vi "Read Started.vi"(8 "error in (no error)":errorcluster, 11 "MQTT_Base in":refnum<class "MQTT_Base.lvclass">) -> (0 "error out":errorcluster, 2 "Started":refnum<notifier>, 3 "MQTT_Base out":refnum<class "MQTT_Base.lvclass">)   [LabVIEW 2013, in "MQTT Base.lvlib" / "MQTT_Base.lvclass"]
uses:
  MQTT_Base.lvclass
  MQTT_Base.lvclass/MQTT_Base.ctl
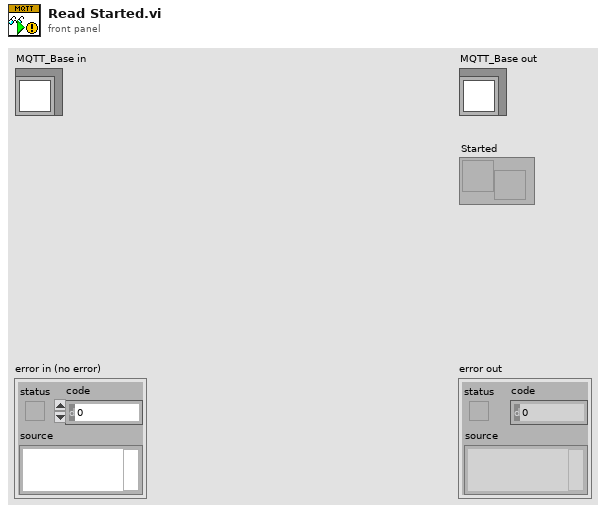
[diagram p1: front panel]
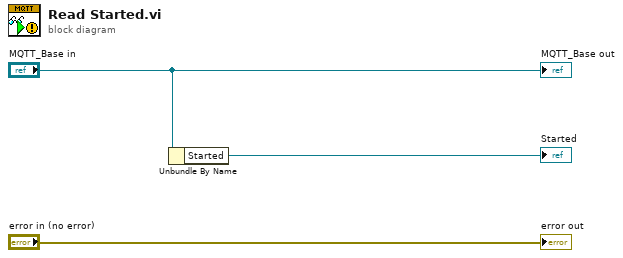
[diagram p0: block diagram]
diagram:
  n1 = Unbundle By Name("MQTT_Base in") -> ("Started"=→"Started":refnum<notifier>)
  "error out" <- "error in (no error)"
  "MQTT_Base out" <- "MQTT_Base in"
